vi "Query.vi"(8 "error in (no error)":errorcluster, 9 "Timeout":i32=10000, 10 "Query":string, 11 "Postgres Connector In":refnum<class "Postgres Connector.lvclass">) -> (0 "error out":errorcluster, 2 "Query Return":T1[](array[typedef]), 3 "Postgres Connector Out":refnum<class "Postgres Connector.lvclass">)   [LabVIEW 2019, in "PG_LIB.lvlib" / "Postgres Connector.lvclass"]
doc: "This VI is used to send a query and retrieve the answer from the PostgreSQL Database"
uses:
  Postgres Connector.lvclass
  Cluster_Return_Of_The_Query.ctl
  Postgres Connector.lvclass/Postgres Connector.ctl
panel:
  out "ReadyForQuery":string
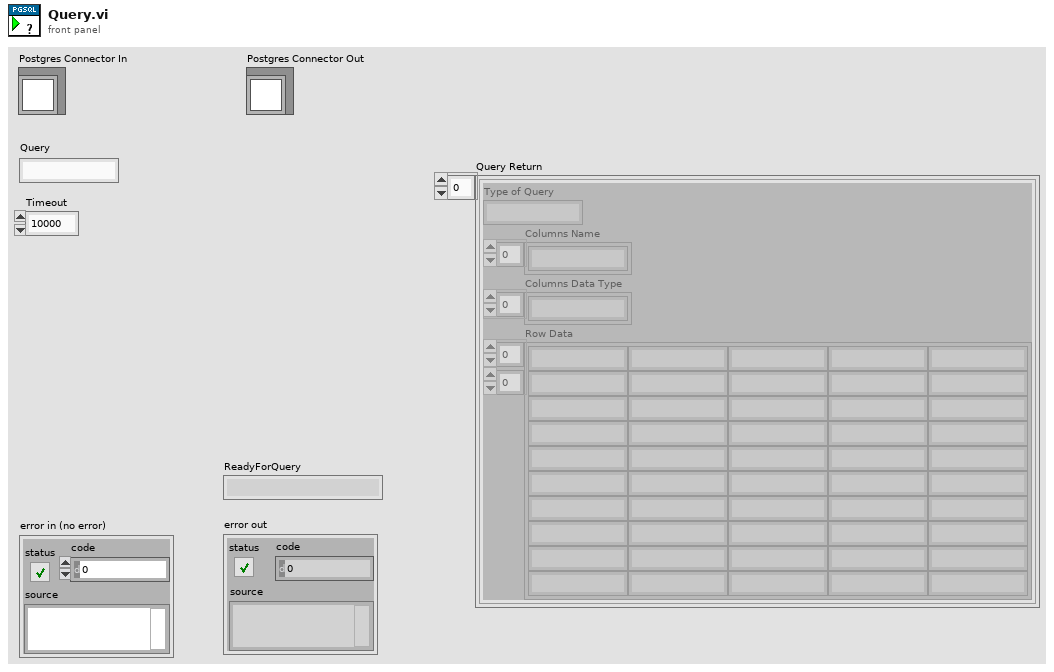
[diagram p1: front panel]
types:
  T1 = typedef "PG_LIB.lvlib/Postgres Connector.lvclass/Cluster_Return_Of_The_Query.ctl" = cluster{"Type of Query":string, "Columns Name":string[], "Columns Data Type":string[], "Row Data":string[][]}
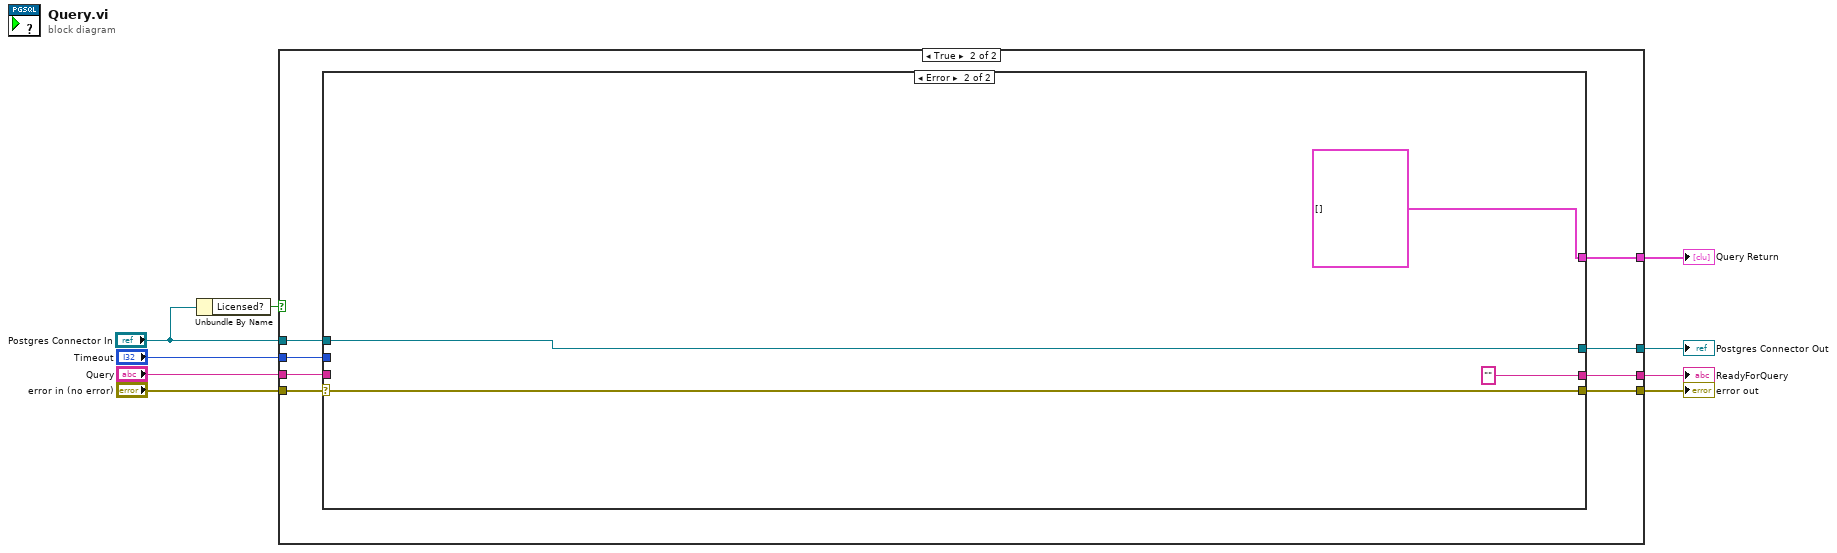
[diagram p0: block diagram]
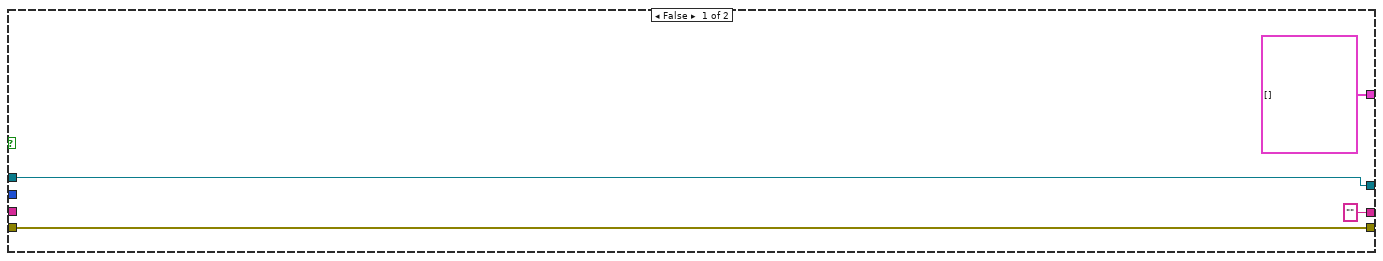
[diagram p2: hidden frame]
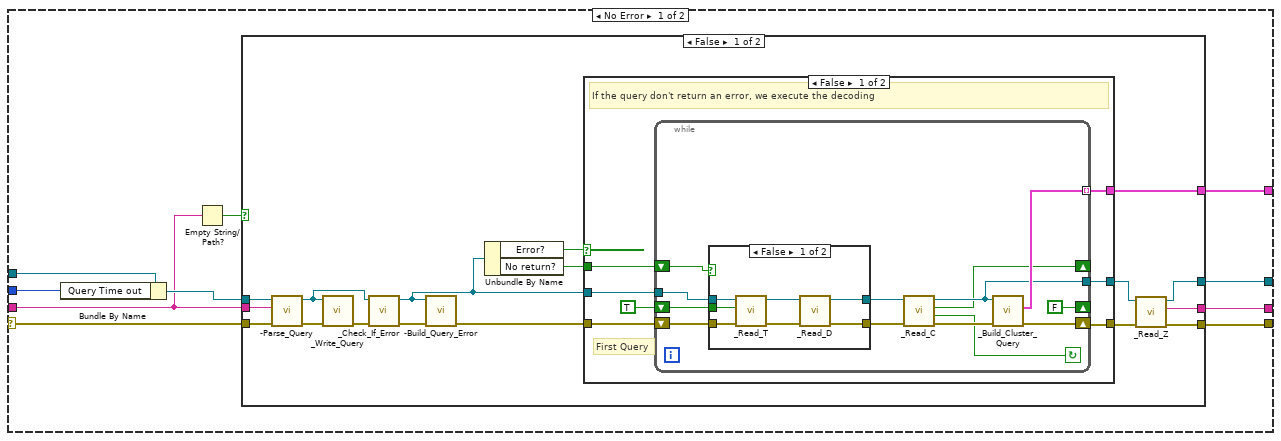
[diagram p3: hidden frame]
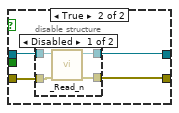
[diagram p4: hidden frame]
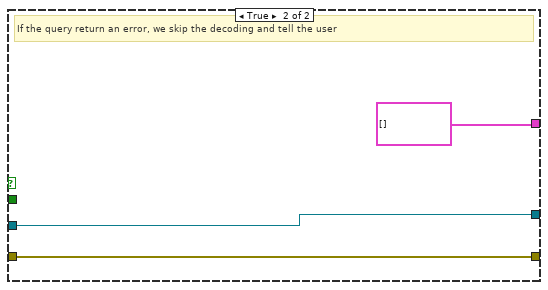
[diagram p6: hidden frame]
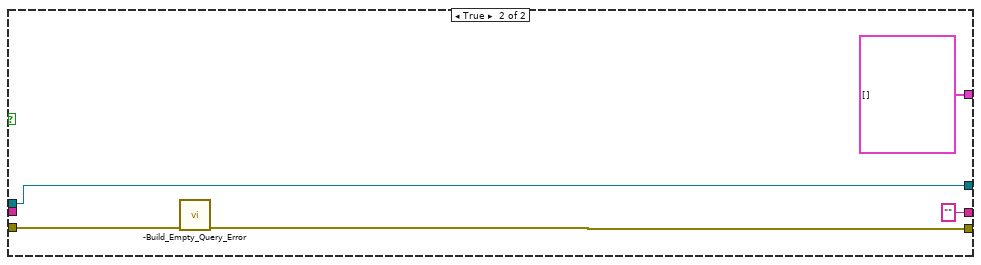
[diagram p7: hidden frame]
diagram:
  n1 = Unbundle By Name("Postgres Connector In") -> ("Licensed?"=w1:bool)
  n2 = case shown="True" w1 {
    tunnel: "error in (no error)" -> [w13 w21]
    tunnel: [w13 w20] -> w8
    tunnel: "Query" -> [_ w19]
    tunnel: "Postgres Connector In" -> [w11 w18]
    tunnel: [w11 w17] -> w6
    tunnel: ["" ("ReadyForQuery") w16] -> w5
    tunnel: [T1[] [] w15] -> w4
    tunnel: "Timeout" -> [_ w14]
    frame False {
    }
    frame True {
      n3 = case shown="Error" w21 {
        selector: w21 -> [w31 w96]
        tunnel: [w24 w96] -> w20
        tunnel: w19 -> [w23 _]
        tunnel: w18 -> [w27 w95]
        tunnel: [w28 w95] -> w17
        tunnel: [w29 "" ("ReadyForQuery")] -> w16
        tunnel: [w30 T1[] []] -> w15
        tunnel: w14 -> [w26 _]
        frame No Error {
          n4 = Bundle By Name(cluster=w27, "Query Time out"=w26) -> (w25:refnum<class "Postgres Connector.lvclass">)
          n5 = Empty String/Path?(string/path=w23) -> (empty?=w22:bool)
          n6 = case shown="False" w22 {
            tunnel: w31 -> [w48 w89]
            tunnel: w23 -> [w47 _]
            tunnel: [w40 T1[] []] -> w30
            tunnel: [w39 "" ("State After Query")] -> w29
            tunnel: [w38 w92] -> w28
            tunnel: w25 -> [w33 w92]
            tunnel: [w32 w88] -> w24
            frame False {
              n7 = call "-Parse_Query.vi"("error in (no error)"=w48, "Query In"=w47, "Postgres Connector In"=w33) -> ("error out"=w46:errorcluster, "Postgres Connector Out"=w44:refnum<class "Postgres Connector.lvclass">)  [unwired: 7 in]
              n8 = call "_Write_Query.vi"("error in (no error)"=w46, "Postgres Connector In"=w44) -> ("error out"=w45:errorcluster)  [unwired: 9 in]
              n9 = call "_Check_If_Error.vi"("error in (no error)"=w45, "Postgres Connector In"=w44) -> ("error out"=w37:errorcluster, "Postgres Connector In 2"=w36:refnum<class "Postgres Connector.lvclass">)  [unwired: 8 in]
              n10 = call "-Build_Query_Error.vi"("error in (no error)"=w37, "Postgres Connector In"=w36) -> ("error out"=w35:errorcluster)  [unwired: 9 in]
              n11 = Unbundle By Name(w36) -> ("Error?"=w42:bool, "No return?"=w34:bool)
              n12 = case shown="False" w42 {
                tunnel: [w51 w87] -> w43
                tunnel: w35 -> [w54 w87]
                tunnel: w36 -> [w53 w86]
                tunnel: [w52 w86] -> w41
                tunnel: [w50 T1[] []] -> w40
                tunnel: w34 -> [w49 _]
                frame False {
                  # "First Query"
                  # "If the query don't return an error, we execute the decoding"
                  n13 = while {
                    tunnel: w53 -> [w62]
                    shift-right: [w67] -> w51
                    shift-left: w54 -> [w66]
                    shift-right: [FALSE] -> _
                    shift-left: TRUE -> [w65]
                    tunnel: [w59] -> w52
                    tunnel: [w60] -> w50 mode=indexing
                    shift-right: [w57] -> _
                    shift-left: w49 -> [w58]
                    stop <- w64 continue-if-true
                    n14 = case shown="False" w58 {
                      tunnel: w66 -> [w73 w78]
                      tunnel: w65 -> [w72 _]
                      tunnel: w62 -> [w71 w75]
                      tunnel: [w69 w77] -> w56
                      tunnel: [w68 w76] -> w61
                      frame False {
                        n15 = call "_Read_T.vi"("error in (no error)"=w73, "First Query?"=w72, "Postgres Connector In"=w71) -> ("error out"=w74:errorcluster, "Postgres Connector Out"=w70:refnum<class "Postgres Connector.lvclass">)  [unwired: 7 in]
                        n16 = call "_Read_D.vi"("error in (no error)"=w74, "Postgres Connector In"=w70) -> ("error out"=w69:errorcluster, "Postgres Connector Out"=w68:refnum<class "Postgres Connector.lvclass">)  [unwired: 8 in]
                      }
                      frame True {
                        n17 = disable-structure shown="Disabled" {
                          disable-tunnel: w78 -> [w82 w83]
                          disable-tunnel: [w81 w83] -> w77
                          disable-tunnel: [w80 w84] -> w76
                          disable-tunnel: w75 -> [w79 w84]
                          frame Disabled {
                            n18 = call "_Read_n.vi"("error in (no error)"=w82, "Postgres Connector In"=w79) -> ("error out"=w81:errorcluster, "Postgres Connector Out"=w80:refnum<class "Postgres Connector.lvclass">)  [unwired: 7 in, 1 out]
                          }
                          frame Enabled {
                          }
                        }
                      }
                    }
                    n19 = call "_Read_C.vi"("error in (no error)"=w56, "Postgres Connector In"=w61) -> ("error out"=w67:errorcluster, "Another Query?"=w64:bool, "No return?"=w57:bool, "Postgres Connector Out"=w59:refnum<class "Postgres Connector.lvclass">)  [unwired: 6 in]
                    n20 = call "_Build_Cluster_Query.vi"("Postgres Connector In"=w59) -> ("Query Return"=w60:T1)  [unwired: 8 in, 2 out]
                  }
                }
                frame True {
                  # "If the query return an error, we skip the decoding and tell the user"
                }
              }
              n21 = call "_Read_Z.vi"("error in (no error)"=w43, "Postgres Connector In"=w41) -> ("error out"=w32:errorcluster, "State After Query"=w39:string, "Postgres Connector Out"=w38:refnum<class "Postgres Connector.lvclass">)  [unwired: 7 in]
            }
            frame True {
              n22 = call "-Build_Empty_Query_Error.vi"("error in (no error)"=w89) -> ("error out"=w88:errorcluster)  [unwired: 10 in]
            }
          }
        }
        frame Error {
        }
      }
    }
  }
  "error out" <- w8
  "Postgres Connector Out" <- w6
  "ReadyForQuery" <- w5
  "Query Return" <- w4
